vi "getLockStatus.vi"(8 "error":errorcluster, 11 "connection ID":refnum<k5>) -> (0 "error out":errorcluster, 1 "authorized":bool, 2 "locked":bool, 3 "connection ID out":refnum<k5>)   [LabVIEW 2016, in "amc_api.lvlib"]
doc: "This function returns if the device is locked and if the current client is authorized to use the device."
uses:
  amc_api.lvlib
panel:
  out "jsonRespIn":string
  out "JSON-response":string="{\"jsonrpc\":\"2.0\",\"method\":\"\",\"params\":[5,1.245,true,\"name\"],\"id\":\"1\"}"
  out "JSON request":string
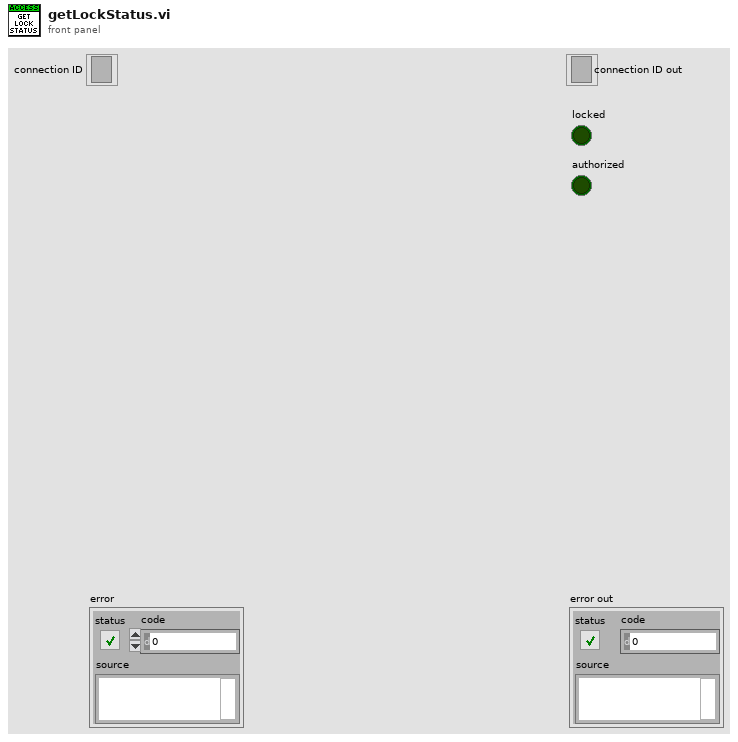
[diagram p1: front panel]
types:
  T1 = cluster{"jsonrpc":string, "method":string, "params":string[], "id":string, "api":i32, "pid":string}
  T2 = enum16{"Standard", "Buffered", "CRLF", "Immediate"}
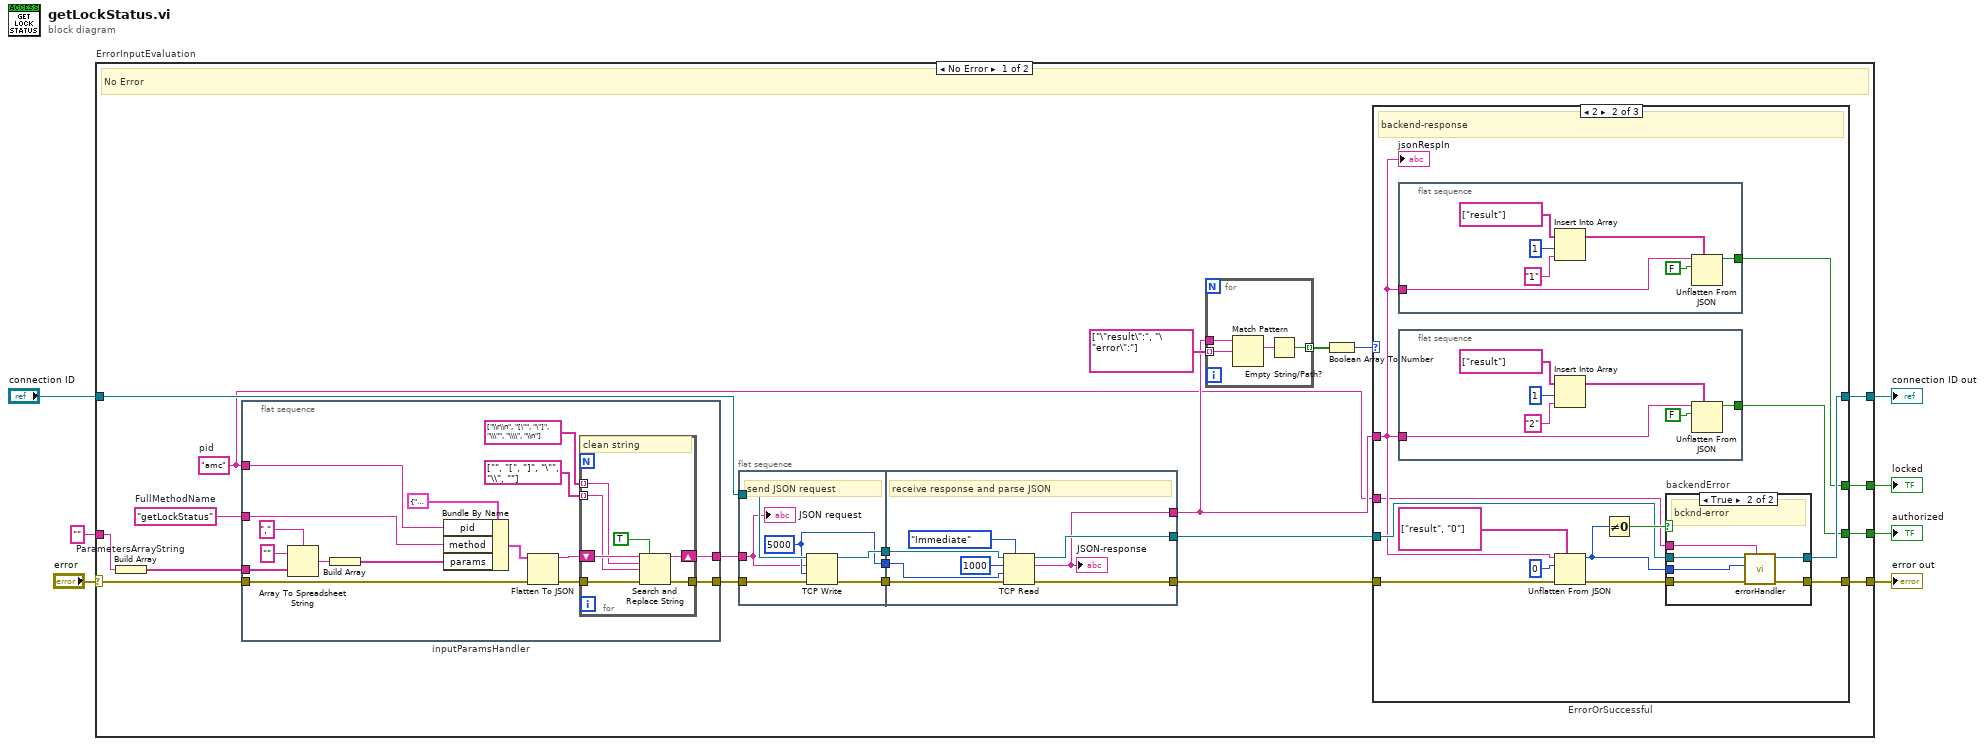
[diagram p0: block diagram]
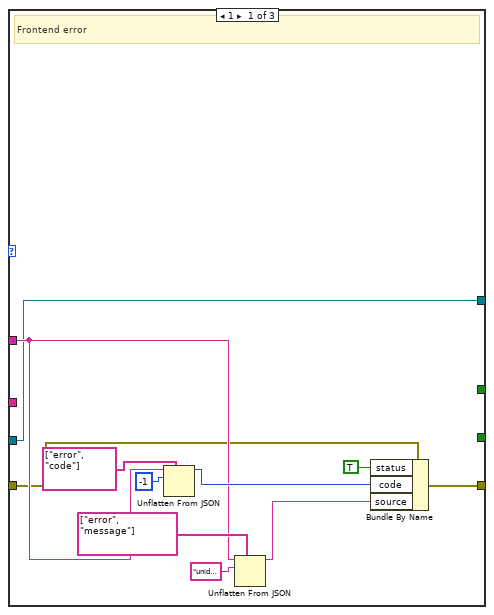
[diagram p2: hidden frame]
diagram:
  n1 = case "ErrorInputEvaluation" shown="No Error" "error" {
    selector: "error" -> [w15 w118]
    tunnel: "connection ID" -> [w25 w119]
    tunnel: [w17 w118] -> w6
    tunnel: [w18 w119] -> w5
    tunnel: "" -> [w10 _]
    tunnel: [w9 _] -> w2
    tunnel: [w8 _] -> w1
    frame No Error {
      w11 = "amc"  # pid
      w16 = "getLockStatus"  # FullMethodName
      # "No Error"
      n2 = Build Array "ParametersArrayString"(w10) -> (w14:string[])
      n3 = flat-sequence "inputParamsHandler" {
        tunnel: [w34] -> w13
        tunnel: w14 -> [w40]
        tunnel: w15 -> [w39]
        tunnel: [w36] -> w12
        tunnel: w16 -> [w30]
        tunnel: w11 -> [w29]
        frame #0 {
          n4 = Array To Spreadsheet String(delimiter (Tab)=",", array=w40, 3:"" ("format string")) -> (spreadsheet string=w42:string)
          n5 = Build Array "Build Array"(w42) -> (w31:string[])
          n6 = Bundle By Name(cluster=T1 {"jsonrpc"="2.0", "method"="com.attocube.amc.res.setRESReadOutFreq", "params"=[], "id"="1", "api"=2, "pid"=""}, "pid"=w29, "method"=w30, "params"=w31) -> (w41:T1)
          n7 = Flatten To JSON(anything=w41, error in (no error)=w39) -> (JSON string=w35:string, 11:w37:errorcluster)  [unwired: 1 in]
          n8 = for {
            tunnel: string[] ["\\r\\n", "[\"", "\"]", "\\\"", "\\\\", "\\n"] ("search string") -> [w48] mode=indexing
            tunnel: string[] ["", "[", "]", "\"", "\\", ""] ("replace string (\"\")") -> [w47] mode=indexing
            shift-right: [w50] -> w34
            shift-left: w35 -> [w49]
            tunnel: w37 -> [w46]
            tunnel: [w45] -> w36
            # "clean string"
            n9 = Search and Replace String(replace all?=TRUE ("replace all? (F)"), input string=w49, search string=w48, replace string=w47, error in=w46) -> (result string=w50:string, error out=w45:errorcluster)  [unwired: 3 in, 2 out]
          }
        }
      }
      n10 = flat-sequence {
        tunnel: w25 -> [w109]
        tunnel: [w107] -> w28
        tunnel: [w108] -> w27
        tunnel: w12 -> [w104]
        tunnel: [w106] -> w26
        tunnel: w13 -> [w105]
        tunnel: [w113] -> w21
        tunnel: w28 -> [w115]
        tunnel: w27 -> [w114]
        tunnel: [w111] -> w20
        tunnel: w26 -> [w112]
        tunnel: [w110] -> w19
        frame #0 {
          w106 = 5000 ("timeout ms (25000)")
          # "send JSON request"
          n11 = TCP Write(connection ID=w109, data in=w105, error in (no error)=w104, 9:w106) -> (connection ID out=w107:refnum<k5>, error out=w108:errorcluster)  [unwired: 1 out]
          "JSON request" <- w105
        }
        frame #1 {
          # "receive response and parse JSON"
          n12 = TCP Read(connection ID=w115, bytes to read=1000, error in (no error)=w114, 7:T2."Immediate" ("mode (standard)"), 9:w112) -> (connection ID out=w113:refnum<k5>, data out=w110:string, error out=w111:errorcluster)
          "JSON-response" <- w110
        }
      }
      n13 = for {
        tunnel: string[] ["\"result\":", "\"error\":"] ("path") -> [w54] mode=indexing
        tunnel: [w52] -> w23 mode=indexing
        tunnel: w19 -> [w55]
        n14 = Match Pattern(string=w55, regular expression=w54) -> (match substring=w53:string)  [unwired: 1 in, 3 out]
        n15 = Empty String/Path?(string/path=w53) -> (empty?=w52:bool)
      }
      n16 = Boolean Array To Number(Boolean array=w23) -> (number=w22:u32)
      n17 = case "ErrorOrSuccessful" shown="2" w22 {
        tunnel: w19 -> [w58 w70 _]
        tunnel: w21 -> [w56 w73 w103]
        tunnel: [w56 w72 w103] -> w18
        tunnel: [w59 w71 w102] -> w17
        tunnel: w20 -> [w57 w74 w102]
        tunnel: w11 -> [_ w69 _]
        tunnel: [_ w68 _] -> w9
        tunnel: [_ w67 _] -> w8
        frame 1 {
          # "Frontend error"
          n18 = Unflatten From JSON(path=string[] ["error", "code"], JSON string=w58, type and defaults=-1) -> (value=w65:i32)  [unwired: 4 in, 1 out]
          n19 = Unflatten From JSON(path=string[] ["error", "message"], JSON string=w58, type and defaults="unidentified error") -> (value=w66:string)  [unwired: 4 in, 1 out]
          n20 = Bundle By Name(cluster=w57, "status"=TRUE, "code"=w65, "source"=w66) -> (w59:errorcluster)
        }
        frame 2 {
          # "backend-response"
          n21 = flat-sequence "out_bool" {
            tunnel: w70 -> [w92]
            tunnel: [w87] -> w68
            frame #0 {
              n22 = Insert Into Array "Insert Into Array"(array=string[] ["result"] ("path"), index=1, new element="1" ("idx")) -> (w89:string[])
              n23 = Unflatten From JSON(path=w89, JSON string=w92, type and defaults=FALSE) -> (value=w87:bool)  [unwired: 4 in, 1 out]
            }
          }
          n24 = flat-sequence "out_bool" {
            tunnel: w70 -> [w85]
            tunnel: [w80] -> w67
            frame #0 {
              n25 = Insert Into Array "Insert Into Array"(array=string[] ["result"] ("path"), index=1, new element="2" ("idx")) -> (w82:string[])
              n26 = Unflatten From JSON(path=w82, JSON string=w85, type and defaults=FALSE) -> (value=w80:bool)  [unwired: 4 in, 1 out]
            }
          }
          n27 = Unflatten From JSON(path=string[] ["result", "0"], JSON string=w70, type and defaults=0, error in (no error)=w74) -> (value=w79:i32, error out=w77:errorcluster)  [unwired: 3 in]
          n28 = Not Equal To 0?(x=w79) -> (x != 0?=w78:bool)
          n29 = case "backendError" shown="True" w78 {
            tunnel: w79 -> [_ w101]
            tunnel: w77 -> [w95 w100]
            tunnel: [w94 w99] -> w72
            tunnel: [w95 w98] -> w71
            tunnel: w73 -> [w94 w97]
            tunnel: w69 -> [_ w96]
            frame False {
              # "successful"
            }
            frame True {
              # "bcknd-error"
              n30 = call "errorHandler.vi"("pid"=w96, "error in"=w100, "errNbr"=w101, "connection ID"=w97) -> ("error out 2"=w98:errorcluster, "connection ID out"=w99:refnum<k5>)  [unwired: 6 in]
            }
          }
          "jsonRespIn" <- w70
        }
        frame Default {
          # "NoResponse"
        }
      }
    }
    frame Error {
      # "Error"
    }
  }
  "error out" <- w6
  "connection ID out" <- w5
  "locked" <- w2
  "authorized" <- w1
